vi "Create Client--SubVI.vi"(7 "Client ID":string="BTSMQTTBRIDGE", 8 "error in (no error)":errorcluster, 10 "remote port (1883)":u16=1883, 11 "address (localhost)":string="localhost") -> (0 "error out":errorcluster, 3 "MQTT_Base out":refnum<class "Client.lvclass">)   [LabVIEW 2024, in "MQTTClient.lvlib"]
doc: "<b>Note:</b> This VI was modified by the <b>Validate DQMH Module</b> tool to turn off automatic error handling."
uses:
  MQTTClient.lvlib
  <vilib>/LabVIEW Open Source Project/MQTT Client/Client class/Client.lvclass
  C:/Program Files/National Instruments/LabVIEW 2025/vi.lib/LabVIEW Open Source Project/MQTT Connection/MQTT_Base/Base Class/MQTT_Base.lvclass
  <vilib>/LabVIEW Open Source Project/MQTT Client/Client class/Client.lvclass/Client.ctl
  <vilib>/LabVIEW Open Source Project/MQTT Connection/MQTT_Base/Base Class/MQTT_Base.lvclass/MQTT_Base.ctl
  <vilib>/LabVIEW Open Source Project/Connection/Connection.TCP/Connection.TCP.lvclass
  C:/Program Files/National Instruments/LabVIEW 2025/vi.lib/LabVIEW Open Source Project/Connection/Connection/Connection.lvclass
  <vilib>/LabVIEW Open Source Project/MQTT Control Packets/Control Packets/PUBLISH/PUBLISH.lvclass
  <vilib>/LabVIEW Open Source Project/MQTT Connection/MQTT_Base/Base Class/MQTT_Base.lvclass
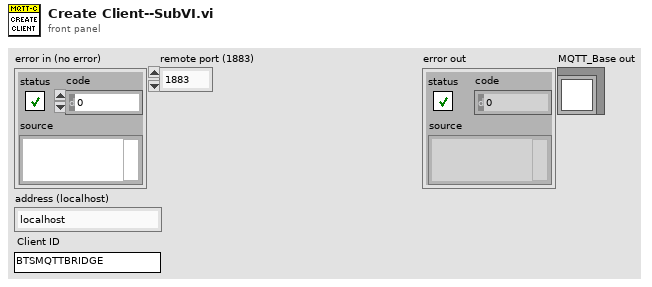
[diagram p1: front panel]
types:
  T1 = typedef "MQTT Client.lvlib/Client.lvclass/Public Events -- cluster.ctl" = cluster{"Connection Status":refnum<user-event>, "Connected":refnum<user-event>, "Application Message":refnum<user-event>}
  T2 = typedef "MQTT Base.lvlib/MQTT_Base.lvclass/Public Events -- cluster.ctl" = cluster{"Stop Event":refnum<user-event>, "Error Event":refnum<user-event>, "Inbound Message":refnum<user-event>}
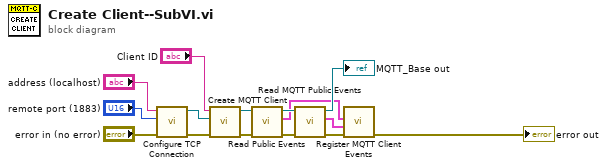
[diagram p0: block diagram]
diagram:
  n1 = call <vilib>:"Configure TCP Connection.vi"("error in (no error)"="error in (no error)", "remote port (80)"="remote port (1883)", "address (localhost)"="address (localhost)") -> ("error out"=w10:errorcluster, "Connection.TCP"=w11:refnum<class "Connection.TCP.lvclass">)  [unwired: 7 in]
  n2 = call <vilib>:"Create MQTT Client.vi"("error in (no error)"=w10, "Connection Configuration"=w11, "ID (empty:generate new)"="Client ID") -> ("error out"=w14:errorcluster, "Client out"=w12:refnum<class "Client.lvclass">)  [unwired: 7 in]
  n3 = call <vilib>:"Read Public Events.vi"("error in (no error)"=w14, "Client in"=w12) -> ("error out"=w15:errorcluster, "Client Public Events"=w1:T1, "Client out"=w13:refnum<class "Client.lvclass">)  [unwired: 7 in]
  n4 = call <vilib>:"Read MQTT Public Events.vi"("error in (no error)"=w15, "MQTT_Base in"=w13) -> ("error out"=w4:errorcluster, "MQTT Public Events"=w2:T2, "MQTT_Base out"=→"MQTT_Base out":refnum<class "Client.lvclass">)  [unwired: 7 in]
  n5 = call "Register MQTT Client Events.vi"("error in"=w4, "MQTT Public Events"=w2, "Client Public Events"=w1) -> ("error out"=→"error out":errorcluster)  [unwired: 8 in]
